vi "version.vi"() -> (2 "version":string="0.0.0.0")   [LabVIEW 2021]
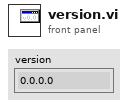
[diagram p1: front panel]
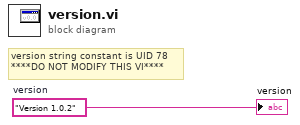
[diagram p0: block diagram]
diagram:
  w1 = "Version 1.0.2"  # version
  # "version string constant is UID 78\n****DO NOT MODIFY THIS VI****"
  "version" <- w1
